vi "TRO_Query.vi"(0 "System no.":i32=1 min=1 max=4 step=1, 2 "TriggerOut to query":string[](array[string]), 3 "All triggers?":bool, 5 "error in":errorcluster) -> (14 "Trigger status?":bool[](array[boolean]), 19 "error out":errorcluster)   [LabVIEW 2020]
doc: "Returns the trigger output mode enable status for the given trigger output lines.\n\nC-702: TriggerOut to query can be 1 to 8.\n\nC-843: TriggerOut to query can be 1 to 4 (4-axis card) or 2 (2-axis card).\n\nC-866: TriggerOut to query can be 1.\n\nC-867, C-877: Check C-867 user manual for available output trigger numbers.\n\nC-413, C-884 , E-871, E-873, E-874 : Check controller user manual for available output trigger numbers.\n\nMercury: TriggerOut to query can be 1 to N (N: number of connected axes, if supported by corresponding Mercury firmware).\n\nMercury_GCS: Check Mercury user manual for available output trigger numbers."
panel:
  # "Returns the trigger output mode enable status for the given \ntrigger output lines."
  # "Query"
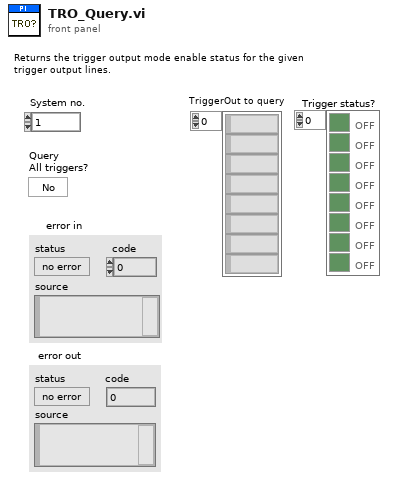
[diagram p1: front panel]
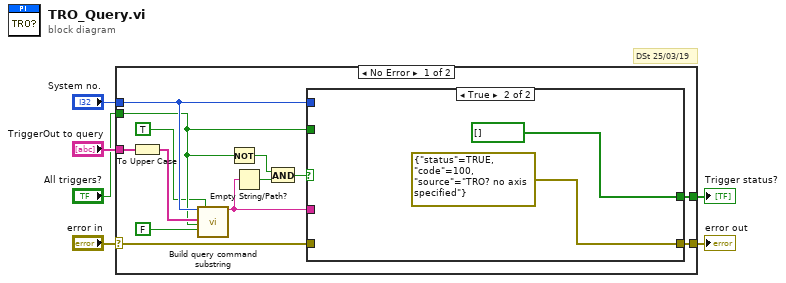
[diagram p0: block diagram]
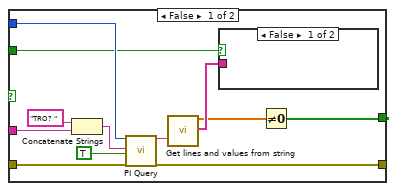
[diagram p2: hidden frame]
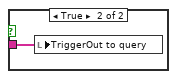
[diagram p3: hidden frame]
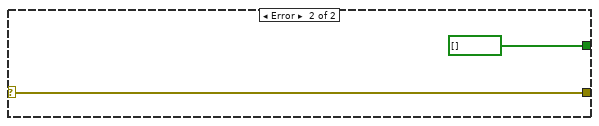
[diagram p4: hidden frame]
diagram:
  # "DSt 25/03/19"
  n1 = case shown="No Error" "error in" {
    selector: "error in" -> [w10 w35]
    tunnel: [w12 bool[] [] ("Booleans")] -> w6
    tunnel: "TriggerOut to query" -> [w19 _]
    tunnel: [w18 w35] -> w4
    tunnel: "System no." -> [w16 _]
    tunnel: "All triggers?" -> [w13 _]
    frame No Error {
      n2 = To Upper Case(1:w19) -> (0:w17:string[])
      n3 = call "Build query command substring.vi"("System no."=w16, "Axes to query in"=w17, "Query\nAll axes?"=w13, "For all axes: use\nAxis identifier?"=FALSE ("For all axes: use\nAxis identifier?"), "With space?"=TRUE) -> ("Command substring"=w8:string)  [unwired: 1 in, 13 out]
      n4 = Not(x=w13) -> (.not. x?=w15:bool)
      n5 = Empty String/Path?(string/path=w8) -> (empty?=w9:bool)
      n6 = And(x=w15, y=w9) -> (x .and. y?=w7:bool)
      n7 = case shown="True" w7 {
        tunnel: [w22 errorcluster {"status"=TRUE, "code"=100, "source"="TRO? no axis specified"} ("error out")] -> w18
        tunnel: w16 -> [w28 _]
        tunnel: w13 -> [w27 _]
        tunnel: [w24 bool[] []] -> w12
        tunnel: w10 -> [w21 _]
        tunnel: w8 -> [w20 _]
        frame False {
          n8 = Concatenate Strings("TRO? ", w20) -> (w29:string)
          n9 = call "PI Query.vi"("System no."=w28, "String to send"=w29, "Attach termination char.?"=TRUE ("Attach Linefeed?"), "error in"=w21) -> ("String read"=w23:string, "error out"=w22:errorcluster)  [unwired: 3 in, 11 out]
          n10 = call "Get lines and values from string.vi"("Input string"=w23) -> ("Numerical values"=w25:dbl[], "Item name"=w26:string[])  [unwired: 1 in, 16 out]
          n11 = case shown="False" w27 {
            tunnel: w26 -> [_ w32]
            frame False {
            }
            frame True {
              n12 = local write "TriggerOut to query"(w32) -> ()
            }
          }
          n13 = Not Equal To 0?(x=w25) -> (x != 0?=w24:bool[])
        }
        frame True {
        }
      }
    }
    frame Error {
    }
  }
  "error out" <- w4
  "Trigger status?" <- w6
